vi "get_material_parameter.vi"(8 "error in (no error)":errorcluster, 9 "Material number":u8=1 min=1 max=32 step=1, 10 "Material parameter":T1, 11 "VISA resource name":refnum<visa-resource-name>) -> (0 "error out":errorcluster, 2 "Material parameter value":string, 3 "VISA resource name out":refnum<visa-resource-name>)   [LabVIEW 2018]
doc: "Set the density of a material."
uses:
  Low Level/material_parameter_enum.ctl
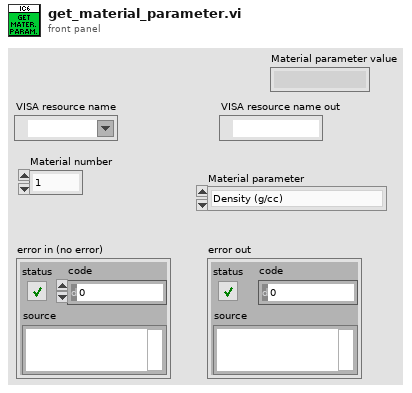
[diagram p1: front panel]
types:
  T1 = typedef "material_parameter_enum.ctl" = enum16{"Density (g/cc)", "Z-Ratio", "Master Tooling (%)", "Control Loop", "Process Gain (A/s/%)", "Time Constant (s)", "Dead Time (s)", "Source", "Maximum Power (%)", "Minimum Power (%)", "Max Power Option", "PreCond Soak Power (%)", "PreCond Rise Time (s) (mm:ss)", "PreCond Soak Time (s) (mm:ss)", "Soak Power 1 (%)", "Rise Time 1 (s) (mm:ss)", "Soak Time 1 (s) (mm:ss)", "Soak Power 2 (%)", "Rise Time 2 (s) (mm:ss)", "Soak Time 2 (s) (mm:ss)", "Auto Soak 2", "Dep After Pre-Dep", "Delay Option", "Control Delay Time (s) (mm:ss)", "Shutter Delay Accur (%)", "Transfer Sensor", "Transfer Tooling (%)", "Feed Power (%)", "Feed Ramp Time (s) (mm:ss)", "Feed Time (s) (mm:ss)", "Idle Power (%)", "Idle Ramp Time (s) (mm:ss)", "Rate (A/s)", "Time Limit (s) (mm:ss)", "Rate Filter Time (s)", "Time Power Avg Time (minutes)", "Ion Assist Deposit", "On Final Thickness", "Ramp 1 Rate (A/s)", "Start Ramp 1 (kA)", "Ramp 1 Time (s) (mm:ss)", "Ramp 2 Rate (A/s)", "Start Ramp 2 (kA)", "Ramp 2 Time (s) (mm:ss)", "RateWatcher Option", "RateWatcher Time (s) (mm:ss)", "RateWatcher Accuracy (%)", "Multipoint", "Aggregate Multiplier", "Sensor 1 Failure Action", "Sensor 2 Failure Action", "Sensor 3 Failure Action", "Sensor 4 Failure Action", "Sensor 5 Failure Action", "Sensor 6 Failure Action", "Sensor 7 Failure Action", "Sensor 8 Failure Action", "Sensor 1 Failure Trigger", "Sensor 2 Failure Trigger", "Sensor 3 Failure Trigger", "Sensor 4 Failure Trigger", "Sensor 5 Failure Trigger", "Sensor 6 Failure Trigger", "Sensor 7 Failure Trigger", "Sensor 8 Failure Trigger", "Sensor 1 Weight (%)", "Sensor 2 Weight (%)", "Sensor 3 Weight (%)", "Sensor 4 Weight (%)", "Sensor 5 Weight (%)", "Sensor 6 Weight (%)", "Sensor 7 Weight (%)", "Sensor 8 Weight (%)", "Sensor 1 Tooling (%)", "Sensor 2 Tooling (%)", "Sensor 3 Tooling (%)", "Sensor 4 Tooling (%)", "Sensor 5 Tooling (%)", "Sensor 6 Tooling (%)", "Sensor 7 Tooling (%)", "Sensor 8 Tooling (%)", "Sensor 1 CrystalTwo Tooling (%)", "Sensor 2 CrystalTwo Tooling (%)", "Sensor 3 CrystalTwo Tooling (%)", "Sensor 4 CrystalTwo Tooling (%)", "Sensor 5 CrystalTwo Tooling (%)", "Sensor 6 CrystalTwo Tooling (%)", "Sensor 7 CrystalTwo Tooling (%)", "Sensor 8 CrystalTwo Tooling (%)", "Sensor 1 Cal Thickness (kA)", "Sensor 2 Cal Thickness (kA)", "Sensor 3 Cal Thickness (kA)", "Sensor 4 Cal Thickness (kA)", "Sensor 5 Cal Thickness (kA)", "Sensor 6 Cal Thickness (kA)", "Sensor 7 Cal Thickness (kA)", "Sensor 8 Cal Thickness (kA)", "Sensor 1 Xtal Position First", "Sensor 2 Xtal Position First", "Sensor 3 Xtal Position First", "Sensor 4 Xtal Position First", "Sensor 5 Xtal Position First", "Sensor 6 Xtal Position First", "Sensor 7 Xtal Position First", "Sensor 8 Xtal Position First", "Sensor 1 Xtal Position Last", "Sensor 2 Xtal Position Last", "Sensor 3 Xtal Position Last", "Sensor 4 Xtal Position Last", "Sensor 5 Xtal Position Last", "Sensor 6 Xtal Position Last", "Sensor 7 Xtal Position Last", "Sensor 8 Xtal Position Last", "Sensor", "Failure Action", "CrystalTwo Tooling (%)", "Xtal Position First", "Xtal Position Last", "Backup Sensor", "Backup Tooling (%)", "Quality Percent (%)", "Quality Counts", "Stability Single (Hz)", "Stability Total (Hz)", "Recorder Output", "Recorder Function", "Recorder Range"}
  T2 = enum16{"Source", "General", "Input name", "Process name", "Logic", "Material", "Material name", "Output name", "Process", "Sensor", "Output type", "User message", "Layer", ""}
  T3 = enum16{"Hello", "Query", "Remote action", "Status", "Update"}
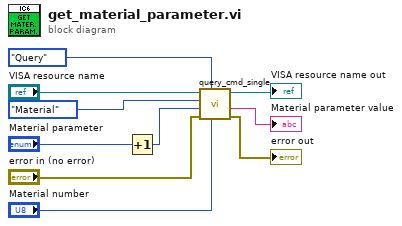
[diagram p0: block diagram]
diagram:
  n1 = Increment(x="Material parameter") -> (x+1=w1:T1)
  n2 = call "query_cmd_single.vi"("Parameter"="Material number", "Command group"=T3."Query", "error in (no error)"="error in (no error)", "Command ID"=w1, "Command subgroup"=T2."Material", "VISA resource name"="VISA resource name") -> ("error out"=→"error out":errorcluster, "formatted response"=→"Material parameter value":string, "VISA resource name out"=→"VISA resource name out":refnum<visa-resource-name>)  [unwired: 1 in, 2 out]
